vi "SetPosition.vi"(8 "error in (no error)":errorcluster, 9 "Y":i16, 10 "X":i16, 11 "RT_Sprite in":refnum<class "RT_Sprite.lvclass">) -> (0 "error out":errorcluster, 3 "RT_Sprite out":refnum<class "RT_Sprite.lvclass">)   [LabVIEW 2019, in "RT_Game.lvlib" / "RT_Sprite.lvclass"]
uses:
  RT_Sprite.lvclass
  C:/Users/FreshBob/Dropbox/VIs/myRIO_GameConsole/RT/RT_Game/GameObject/GameObject.lvclass
  GameObject/GameObject.lvclass/GameObject.ctl
  GameObject/Write position.vi
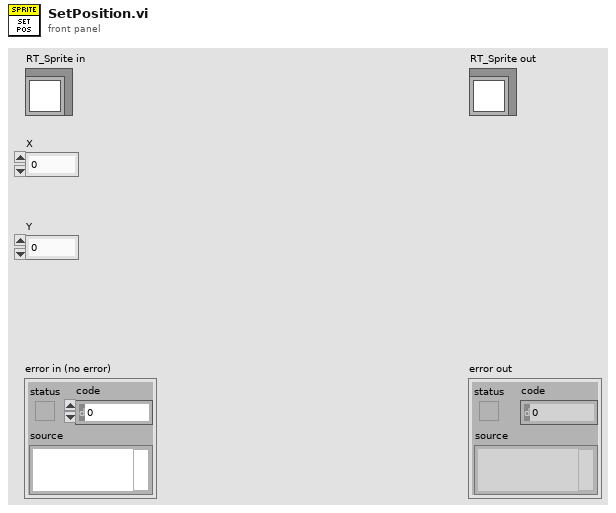
[diagram p1: front panel]
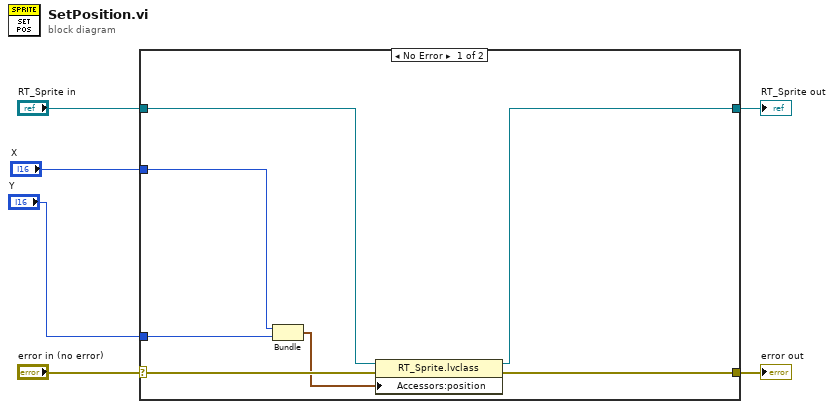
[diagram p0: block diagram]
diagram:
  n1 = case shown="No Error" "error in (no error)" {
    selector: "error in (no error)" -> [w13 w15]
    tunnel: [w12 w15] -> w5
    tunnel: [w10 w14] -> w3
    tunnel: "RT_Sprite in" -> [w11 w14]
    tunnel: "X" -> [w8 _]
    tunnel: "Y" -> [w7 _]
    frame No Error {
      n2 = Bundle("X"=w8, "Y"=w7) -> (w9:cluster{"X":i16, "Y":i16})  [unwired: 1 in]
      n3 = property class="RT_Sprite.lvclass"(reference=w11, error in=w13, "Accessors:position"=w9) -> (reference out=w10:refnum<class "RT_Sprite.lvclass">, error out=w12:errorcluster)
    }
    frame Error {
    }
  }
  "error out" <- w5
  "RT_Sprite out" <- w3
